vi "ExposeMakeEventStreamNameFromIDAndCategory.vi"(9 "Category":string, 11 "ID":string) -> (3 "StreamName":string)   [LabVIEW 2017]
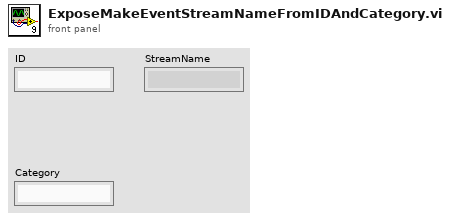
[diagram p1: front panel]
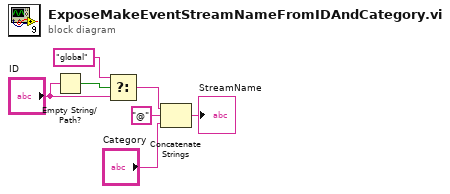
[diagram p0: block diagram]
diagram:
  n1 = Empty String/Path?(string/path="ID") -> (empty?=w4:bool)
  n2 = Select(t="global", s=w4, f="ID") -> (s? t:f=w1:string)
  n3 = Concatenate Strings(w1, "@" ("string"), "Category") -> (→"StreamName":string)
